vi "PLAYGROUND.vi"() -> ()   [LabVIEW 2018]
uses:
  Pressure_Cluster.ctl
panel:
  out "x .or. y?":bool
  out "size(s)":i32
  out "Array 2":string[](array[string])
  in  "Pressure Cluster 2":T1
  out "Ring":u16(ring) items=["Pressure", "Pressure ENG2", "Pressure ENG3", "Pressure ENG4"]
  out "Array":string[](array[string])
  in  "Pressure Cluster":T1
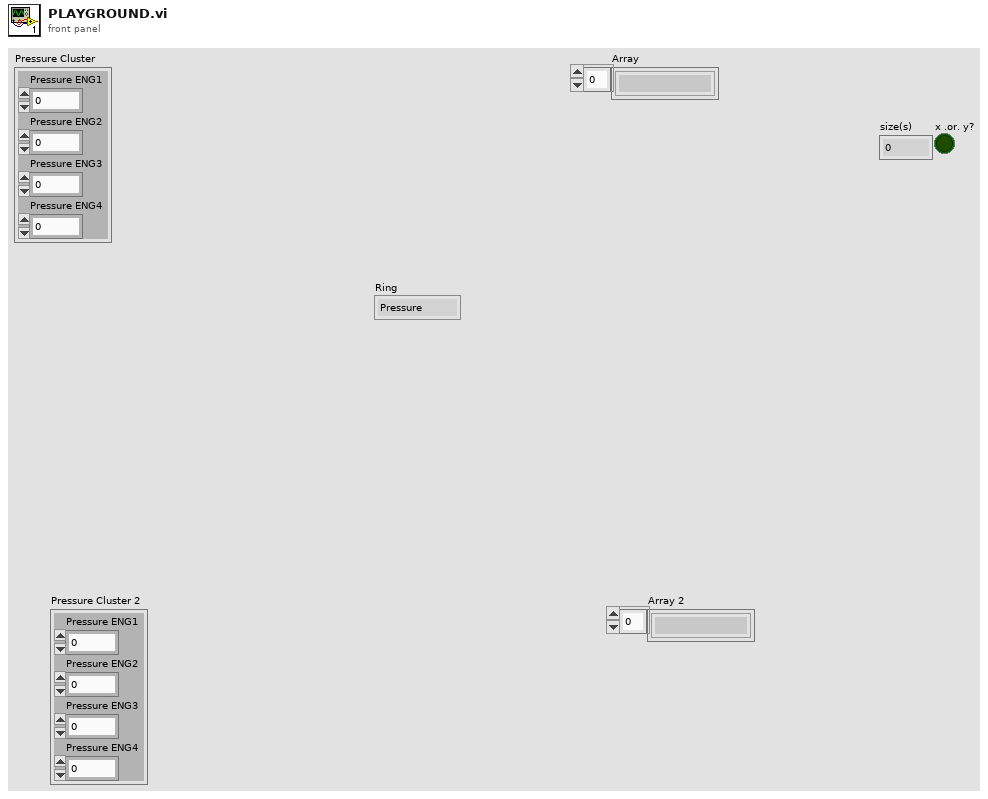
[diagram p1: front panel]
types:
  T1 = typedef "Pressure_Cluster.ctl" = cluster{"Pressure ENG1":dbl, "Pressure ENG2":dbl, "Pressure ENG3":dbl, "Pressure ENG4":dbl}
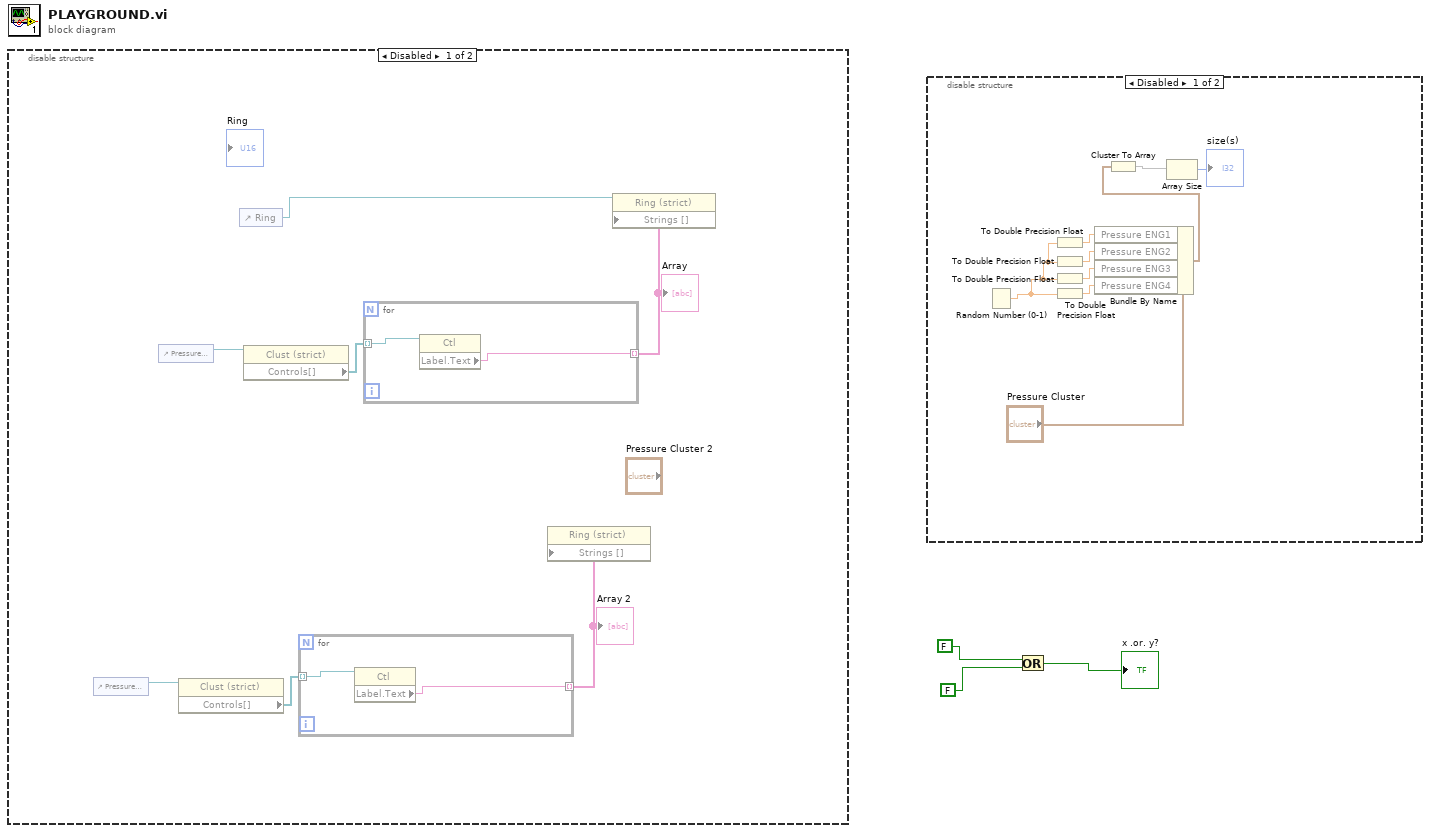
[diagram p0: block diagram]
diagram:
  n1 = disable-structure shown="Disabled" {
    frame Disabled {
      n2 = control-ref of="Pressure Cluster 2"() -> (w6:refnum<vi>)
      n3 = control-ref of="Pressure Cluster"() -> (w10:refnum<vi>)
      n4 = property class="Clust (strict)"(reference=w6) -> ("Controls[]"=w5:refnum<vi>[])  [unwired: 1 in, 2 out]
      n5 = control-ref of="Ring"() -> (w8:refnum<vi>)
      n6 = property class="Clust (strict)"(reference=w10) -> ("Controls[]"=w9:refnum<vi>[])  [unwired: 1 in, 2 out]
      n7 = for {
        tunnel: w5 -> [w12] mode=indexing
        tunnel: [w11] -> w4 mode=indexing
        n8 = property class="Ctl"(reference=w12) -> ("Label.Text"=w11:string)  [unwired: 1 in, 2 out]
      }
      "Array 2" <- w4
      n9 = for {
        tunnel: w9 -> [w14] mode=indexing
        tunnel: [w13] -> w7 mode=indexing
        n10 = property class="Ctl"(reference=w14) -> ("Label.Text"=w13:string)  [unwired: 1 in, 2 out]
      }
      "Array" <- w7
      n11 = property class="Ring (strict)"("Strings []"=w4) -> ()  [unwired: 2 in, 2 out]
      n12 = property class="Ring (strict)"(reference=w8, "Strings []"=w7) -> ()  [unwired: 1 in, 2 out]
    }
    frame Enabled {
    }
  }
  n13 = disable-structure shown="Disabled" {
    frame Disabled {
      n14 = Random Number (0-1)() -> (number: 0 to 1=w17:dbl)
      n15 = To Double Precision Float(number=w17) -> (double precision float=w23:dbl)
      n16 = To Double Precision Float(number=w17) -> (double precision float=w22:dbl)
      n17 = To Double Precision Float(number=w17) -> (double precision float=w21:dbl)
      n18 = To Double Precision Float(number=w17) -> (double precision float=w20:dbl)
      n19 = Bundle By Name(cluster="Pressure Cluster", "Pressure ENG1"=w23, "Pressure ENG2"=w22, "Pressure ENG3"=w21, "Pressure ENG4"=w20) -> (w19:T1)
      n20 = Cluster To Array(cluster=w19) -> (array=w18:dbl[])
      n21 = Array Size(array=w18) -> (size(s)=→"size(s)":i32)
    }
    frame Enabled {
    }
  }
  n22 = Or(x=FALSE, y=FALSE) -> (x .or. y?=→"x .or. y?":bool)
